vi "FoundInstruments.vi"(8 "error in (no error)":errorcluster, 10 "FoundInstruments":T1, 11 "InterferometryUI in":refnum<class "InterferometryUI.lvclass">) -> (0 "error out":errorcluster, 3 "InterferometryUI out":refnum<class "InterferometryUI.lvclass">)   [LabVIEW 2023, in "InterferometryUI.lvlib" / "InterferometryUI.lvclass"]
uses:
  InterferometryUI.lvclass
  typedefs/instrumentType.ctl
  typedefs/typedefs.lvlib
  <vilib>/ActorFramework/Message Enqueuer/Message Enqueuer.lvclass
  SinglePhoton_UI/typedefs/FoundInstruments.ctl
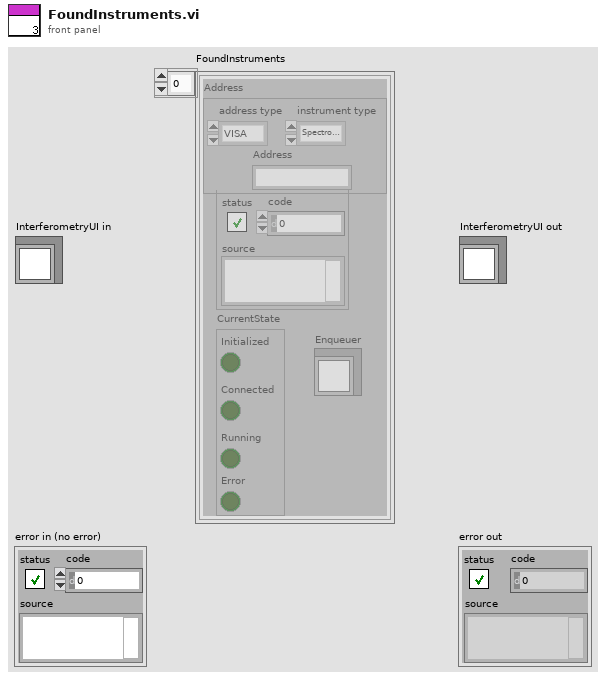
[diagram p1: front panel]
types:
  T1 = typedef "typedefs.lvlib/FoundInstruments.ctl" = cluster{"Instr Error":errorcluster, "Address":cluster{"address type":enum16{"VISA", "Index"}, "Address":string, "instrument type":T2}, "CurrentState":cluster{"Initialized":bool, "Connected":bool, "Running":bool, "Error":bool}, "Enqueuer":refnum<class "Message Enqueuer.lvclass">}[]
  T2 = typedef "typedefs.lvlib/instrumentType.ctl" = enum16{"Spectrometer", "Camera", "Stepper", "Piezo", "SLM"}
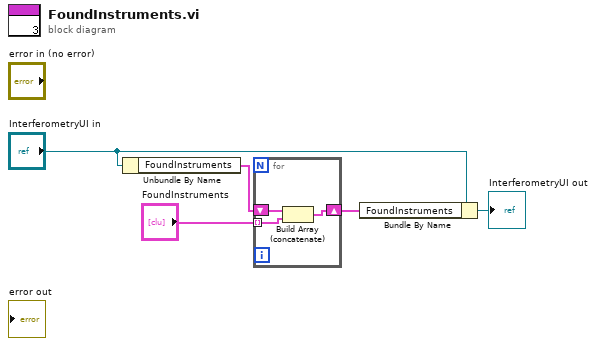
[diagram p0: block diagram]
diagram:
  n1 = Unbundle By Name("InterferometryUI in") -> ("FoundInstruments"=w4:T1)
  n2 = for {
    shift-right: [w7] -> w2
    shift-left: w4 -> [w8]
    tunnel: "FoundInstruments" -> [w6] mode=indexing
    n3 = Build Array (concatenate)(w8, w6) -> (w7:T1)
  }
  n4 = Bundle By Name(cluster="InterferometryUI in", "FoundInstruments"=w2) -> (→"InterferometryUI out":refnum<class "InterferometryUI.lvclass">)
